vi "Clock 2012 NIVerified.vi"() -> ()   [LabVIEW 2019]
doc: "This is an example VI which uses four guages to show an analogue clock. The timestamp is retrieved from the computer, and analysed every 100ms. Values for hour, minute, and seconds are single precision, and the clock is updated every 100ms. This gives the impression of constantly flowing dials."
panel:
  out "Second":sgl(knob) scale=0.0..60.0
  out "Minute":sgl(knob) scale=0.0..60.0
  out "Hour":sgl(knob) scale=0.0..12.0
  out "Dial":sgl(knob) scale=0.0..12.0
  # "Overview: This example shows how to use customized gauges on the front panel to create an analogue clock. \nRequirements: LabVIEW 2012 (or compatible)\nInstructions:\nRun the VI to see it working."
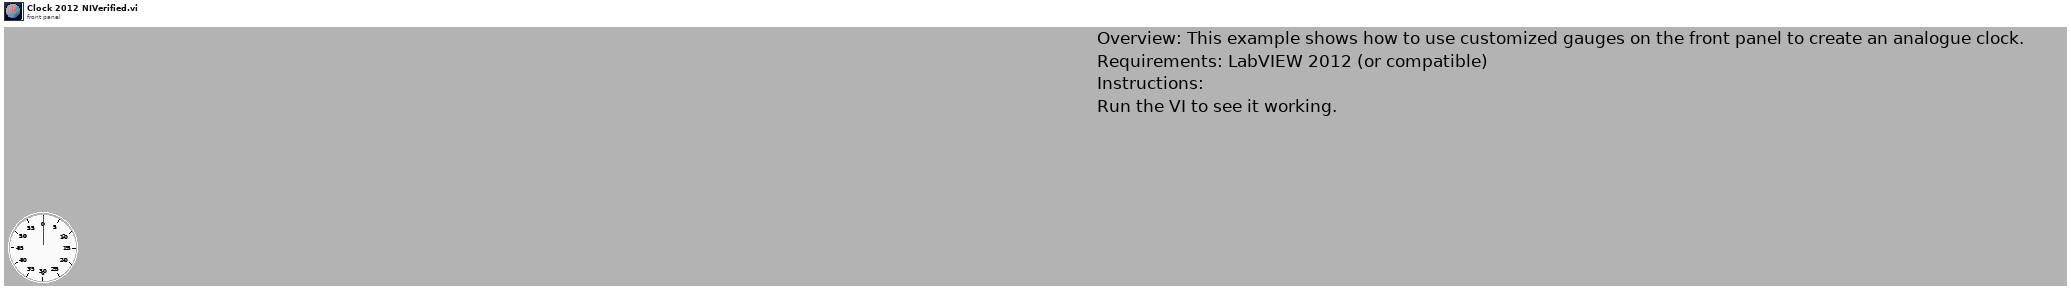
[diagram p1: front panel]
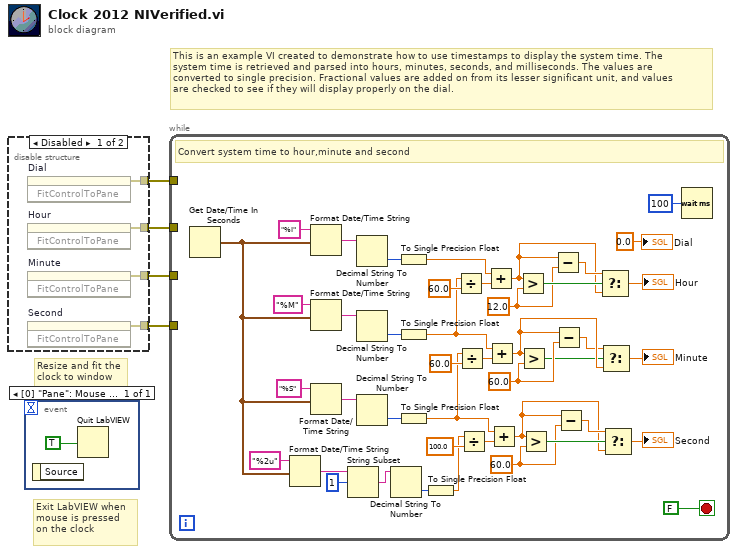
[diagram p0: block diagram]
diagram:
  # "Exit LabVIEW when\nmouse is pressed\non the clock"
  # "Resize and fit the\nclock to window"
  # "This is an example VI created to demonstrate how to use timestamps to display the system time. The \nsystem time is retrieved and parsed into hours, minutes, seconds, and milliseconds. The values are\nconverted to single precision. Fractional values are added on from its lesser significant unit, and values\nare checked to see if they will display properly on the dial."
  n1 = disable-structure shown="Disabled" {
    disable-tunnel: [w8 _] -> w4
    disable-tunnel: [w7 _] -> w3
    disable-tunnel: [w6 _] -> w2
    disable-tunnel: [w5 _] -> w1
    frame Disabled {
      n2 = invoke on="Dial" class="Knob (strict)" method="FitControlToPane"() -> (error out=w8:errorcluster)  [unwired: 3 in, 2 out]
      n3 = invoke on="Hour" class="Knob (strict)" method="FitControlToPane"() -> (error out=w7:errorcluster)  [unwired: 3 in, 2 out]
      n4 = invoke on="Minute" class="Knob (strict)" method="FitControlToPane"() -> (error out=w6:errorcluster)  [unwired: 3 in, 2 out]
      n5 = invoke on="Second" class="Knob (strict)" method="FitControlToPane"() -> (error out=w5:errorcluster)  [unwired: 3 in, 2 out]
    }
    frame Enabled {
    }
  }
  n6 = event shown="[0] \"Pane\": Mouse Down" {
    selector: _ -> [_]
    dyn-events: _ -> [_]
    timeout: _ -> [_]
    event Mouse Down {
      n7 = event-data() -> ()  [unwired: 1 in, 1 out]
      n8 = Quit LabVIEW(quit? (T)=TRUE) -> ()
    }
  }
  n9 = while {
    tunnel: w4 -> [_]
    tunnel: w3 -> [_]
    tunnel: w2 -> [_]
    tunnel: w1 -> [_]
    stop <- FALSE stop-if-true
    w16 = sgl 60.0 ("y")
    w31 = sgl 60.0 ("y")
    w36 = sgl 12.0 ("y")
    # "Convert system time to hour,minute and second"
    n10 = Get Date/Time In Seconds() -> (seconds since 1Jan1904=w24:timestamp)
    n11 = Format Date/Time String(time format string (%c)="%2u", seconds (now)=w24) -> (date/time string=w23:string)  [unwired: 1 in]
    n12 = Format Date/Time String(time format string (%c)="%I", seconds (now)=w24) -> (date/time string=w48:string)  [unwired: 1 in]
    n13 = Format Date/Time String(time format string (%c)="%M", seconds (now)=w24) -> (date/time string=w45:string)  [unwired: 1 in]
    n14 = Format Date/Time String(time format string (%c)="%S", seconds (now)=w24) -> (date/time string=w43:string)  [unwired: 1 in]
    n15 = String Subset(string=w23, offset (0)=1) -> (substring=w20:string)  [unwired: 1 in]
    n16 = Decimal String To Number(string=w48) -> (number=w47:i32)  [unwired: 2 in, 1 out]
    n17 = Decimal String To Number(string=w45) -> (number=w46:i32)  [unwired: 2 in, 1 out]
    n18 = Decimal String To Number(string=w43) -> (number=w44:i32)  [unwired: 2 in, 1 out]
    n19 = Decimal String To Number(string=w20) -> (number=w21:i32)  [unwired: 2 in, 1 out]
    n20 = To Single Precision Float(number=w47) -> (single precision float=w39:sgl)
    n21 = To Single Precision Float(number=w46) -> (single precision float=w27:sgl)
    n22 = To Single Precision Float(number=w44) -> (single precision float=w13:sgl)
    n23 = To Single Precision Float(number=w21) -> (single precision float=w12:sgl)
    n24 = Divide(x=w27, y=sgl 60.0) -> (x/y=w41:sgl)
    n25 = Divide(x=w13, y=sgl 60.0) -> (x/y=w28:sgl)
    n26 = Divide(x=w12, y=sgl 100.0) -> (x/y=w19:sgl)
    n27 = Add(x=w39, y=w41) -> (x+y=w34:sgl)
    n28 = Add(x=w27, y=w28) -> (x+y=w33:sgl)
    n29 = Add(x=w13, y=w19) -> (x+y=w14:sgl)
    n30 = Greater?(x=w34, y=w36) -> (0:w38:bool)
    n31 = Greater?(x=w33, y=w31) -> (0:w30:bool)
    n32 = Greater?(x=w14, y=w16) -> (0:w17:bool)
    n33 = Subtract(x=w34, y=w36) -> (x-y=w35:sgl)
    n34 = Subtract(x=w33, y=w31) -> (x-y=w32:sgl)
    n35 = Subtract(x=w14, y=w16) -> (x-y=w15:sgl)
    n36 = Select(t=w35, s=w38, f=w34) -> (s? t:f=→"Hour":sgl)
    n37 = Select(t=w32, s=w30, f=w33) -> (s? t:f=→"Minute":sgl)
    n38 = Select(t=w15, s=w17, f=w14) -> (s? t:f=→"Second":sgl)
    n39 = Wait (ms)(milliseconds to wait=u32 100 ("millisecond multiple")) -> ()  [unwired: 1 out]
    "Dial" <- sgl 0.0 ("Dial")
  }
